vi "PCE-Format.vi"(2 "Commande":string, 7 "Arguments":dbl[](array[numeric])) -> (8 "Chaîne formatée":string)   [LabVIEW 2011]
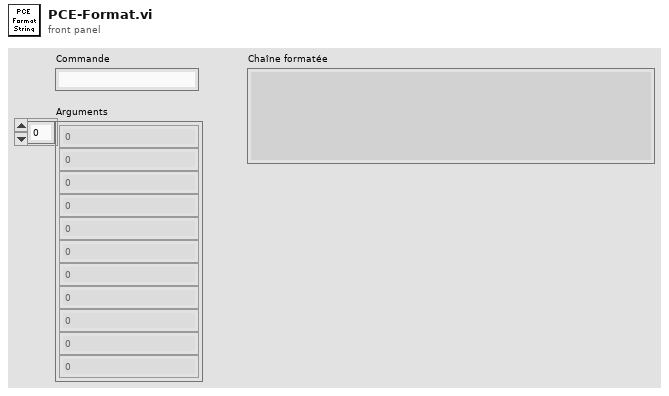
[diagram p1: front panel]
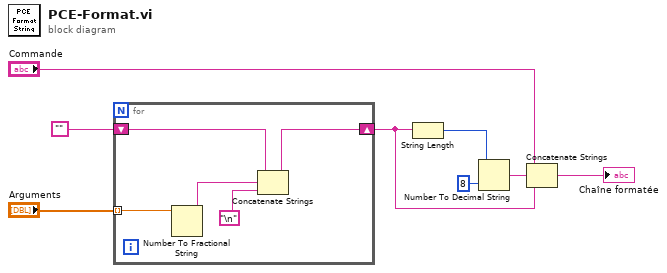
[diagram p0: block diagram]
diagram:
  n1 = for {
    tunnel: "Arguments" -> [w11] mode=indexing
    shift-right: [w12] -> w2
    shift-left: "" -> [w13]
    n2 = Number To Fractional String(number=w11) -> (F-format string=w10:string)  [unwired: 3 in]
    n3 = Concatenate Strings(w13, w10, "\n") -> (w12:string)
  }
  n4 = String Length(string=w2) -> (length=w5:i32)
  n5 = Number To Decimal String(number=w5, width (-)=i16 8) -> (decimal integer string=w4:string)
  n6 = Concatenate Strings("Commande", w4, w2) -> (→"Chaîne formatée":string)
